vi "FilterWaveformByPlot.vi"(8 "error in (no error)":errorcluster, 10 "ListBox in":refnum<vi>, 11 "element":waveform(dbl)[](array[waveform])) -> (0 "error IO":errorcluster, 3 "Array":waveform(dbl)[](array[waveform]))   [LabVIEW 2023]
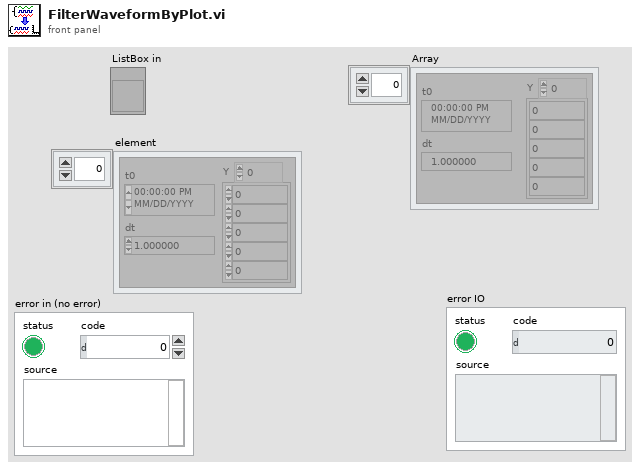
[diagram p1: front panel]
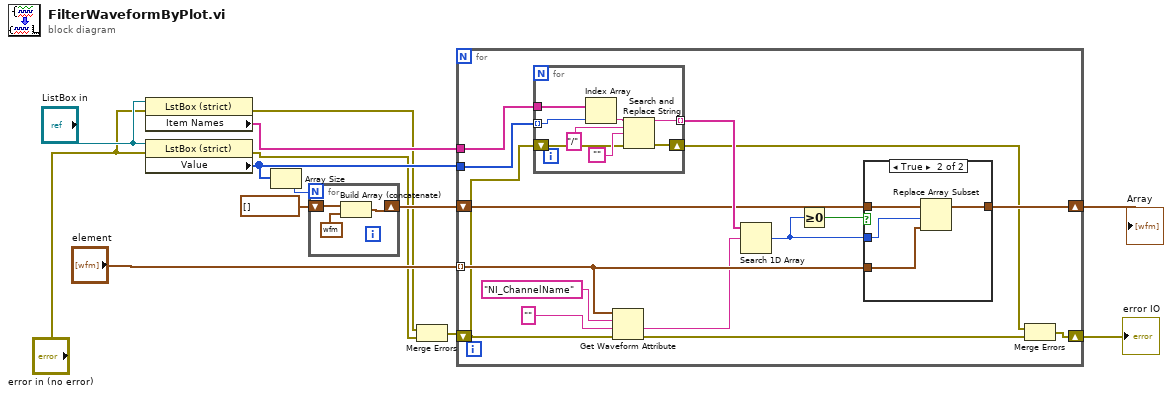
[diagram p0: block diagram]
diagram:
  n1 = property class="LstBox (strict)"(reference="ListBox in", error in="error in (no error)") -> (error out=w3:errorcluster, "Item Names"=w9:string[])  [unwired: 1 out]
  n2 = property class="LstBox (strict)"(reference="ListBox in", error in="error in (no error)") -> (error out=w4:errorcluster, "Value"=w10:i32[])  [unwired: 1 out]
  n3 = Array Size(array=w10) -> (size(s)=w13:i32)
  n4 = for {
    N: w13 -> [_]
    shift-right: [w15] -> w11
    shift-left: waveform(dbl)[] [] -> [w14]
    n5 = Build Array (concatenate)(w14, waveform(dbl) {"t0"=timestamp(0 s since 1904-01-01), "dt"=1.0, "Y"=[]} ("Waveform")) -> (w15:waveform(dbl)[])
  }
  n6 = Merge Errors(w3, w4) -> (w5:errorcluster)
  n7 = for {
    tunnel: "element" -> [w30] mode=indexing
    shift-right: [w24] -> w8
    shift-left: w11 -> [w23]
    tunnel: w9 -> [w22]
    tunnel: w10 -> [w21]
    shift-right: [w18] -> w2
    shift-left: w5 -> [w17]
    n8 = for {
      tunnel: w21 -> [w44] mode=indexing
      tunnel: [w39] -> w29 mode=indexing
      tunnel: w22 -> [w43]
      shift-right: [w38] -> w20
      shift-left: w17 -> [w37]
      n9 = Index Array(array=w43, index=w44) -> (element=w42:string)
      n10 = Search and Replace String(input string=w42, search string="/", replace string="", error in=w37) -> (result string=w39:string, error out=w38:errorcluster)  [unwired: 4 in, 2 out]
    }
    n11 = Get Waveform Attribute(4:w17, 5:"", 6:"NI_ChannelName" ("name"), 7:w30) -> (0:w19:errorcluster, 1:w27:string)  [unwired: 2 out]
    n12 = Search 1D Array(1D array=w29, element=w27) -> (index of element=w25:i32)  [unwired: 1 in]
    n13 = Greater Or Equal To 0?(x=w25) -> (x >= 0?=w26:bool)
    n14 = case shown="True" w26 {
      tunnel: w30 -> [_ w34]
      tunnel: w25 -> [_ w35]
      tunnel: w23 -> [w32 w36]
      tunnel: [w32 w33] -> w24
      frame False {
      }
      frame True {
        n15 = Replace Array Subset(array=w36, new element=w34, index=w35) -> (w33:waveform(dbl)[])
      }
    }
    n16 = Merge Errors(w20, w19) -> (w18:errorcluster)
  }
  "Array" <- w8
  "error IO" <- w2
